vi "Is Name Multiplatform_Allow Multibyte.vi"(8 "error in (no error)":errorcluster, 9 "Replacement":string="-", 10 "name must work for all platforms (F)":bool, 11 "filename":string) -> (0 "error out":errorcluster, 1 "name had problem":bool, 3 "suggested filename":string, 4 "problem description":string)   [LabVIEW 2020, in "NI_Multibyte Utilities.lvlib"]
uses:
  <vilib>/Utility/Multibyte/NI_Multibyte Utilities.lvlib
panel:
  in  "Last Character Windows Warning":string="Windows filenames cannot terminate with the . character."
  in  "Platform Warnings":string[](array[string])=["Windows filenames cannot contain any of these characters: \\ : / * ? \" < > |.", "Macintosh filenames cannot contain the : character.", "Linux filenames cannot contain the / character."]
  in  "Empty filename":string="An empty string is not a valid filename."
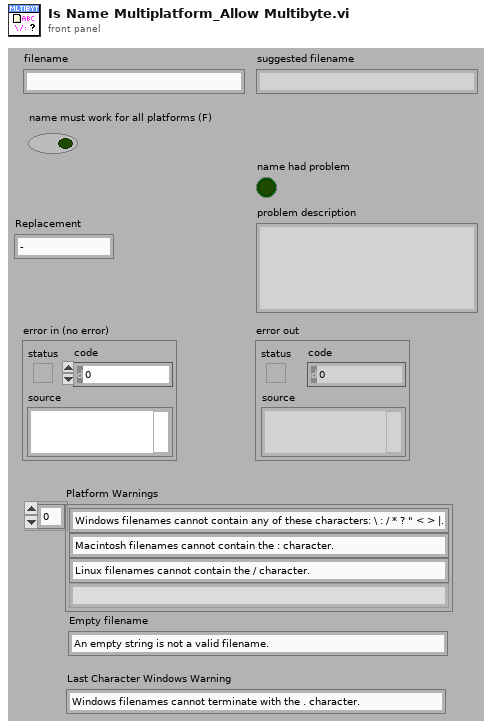
[diagram p1: front panel]
types:
  T1 = cluster{enum32{"invalid OS target", "Mac OS", "Windows 3.1", "Windows 95/NT", "Solaris 1", "Solaris 2", "HP-UX", "PowerMAX", "Linux", "Irix", "Rhapsody", "BeOS", "AIX", "OSF1", "VxWorks", "PharLap", "Carbon", "RTX", "Windows x64", "Linux x64"}[]}[]
  T2 = enum32{"invalid OS target", "Mac OS", "Windows 3.1", "Windows 95/NT", "Solaris 1", "Solaris 2", "HP-UX", "PowerMAX", "Linux", "Irix", "Rhapsody", "BeOS", "AIX", "OSF1", "VxWorks", "PharLap", "Carbon", "RTX", "Windows x64", "Linux x64", "Mac OS X x64"}
  T3 = enum32{"invalid OS target", "Mac OS", "Windows 3.1", "Windows 95/NT", "Solaris 1", "Solaris 2", "HP-UX", "PowerMAX", "Linux", "Irix", "Rhapsody", "BeOS", "AIX", "OSF1", "VxWorks", "PharLap", "Carbon", "RTX", "Windows x64", "Linux x64"}[]
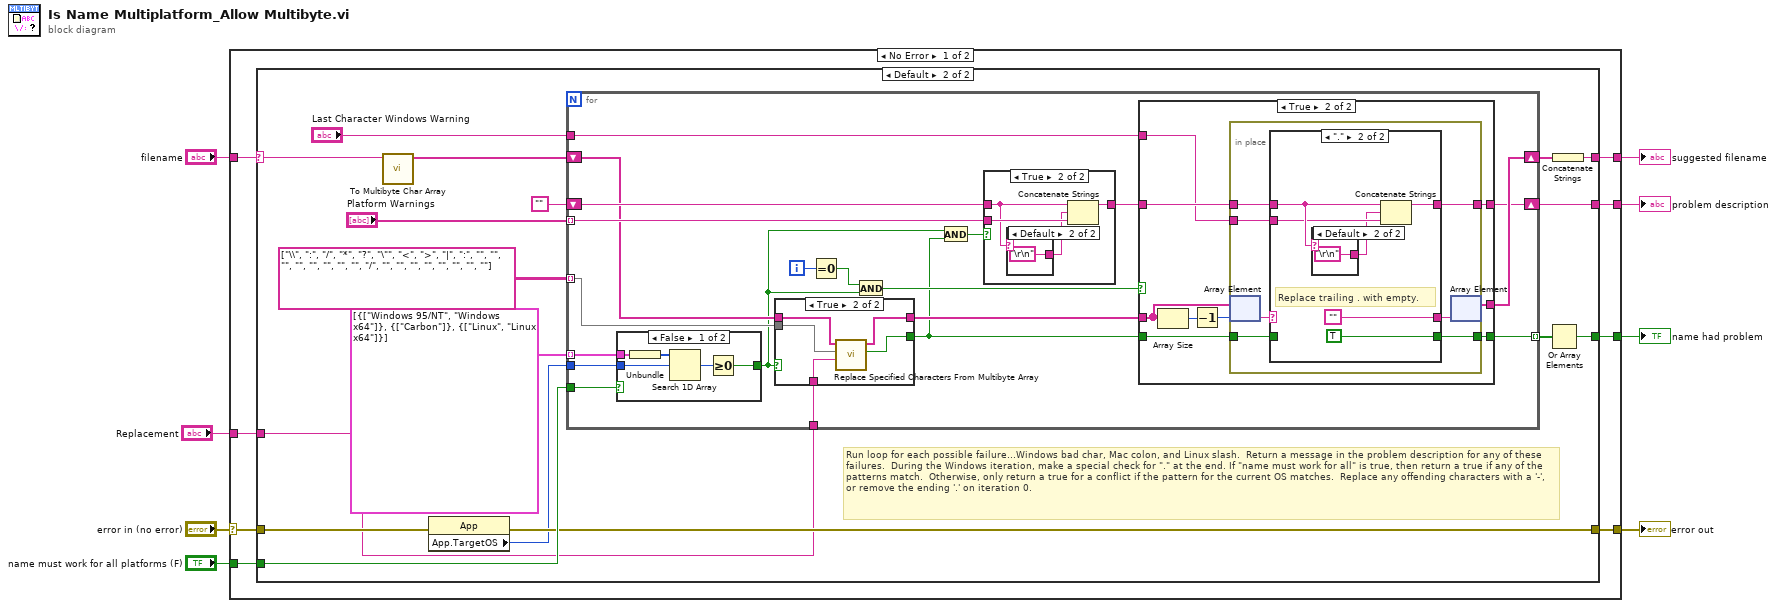
[diagram p0: block diagram]
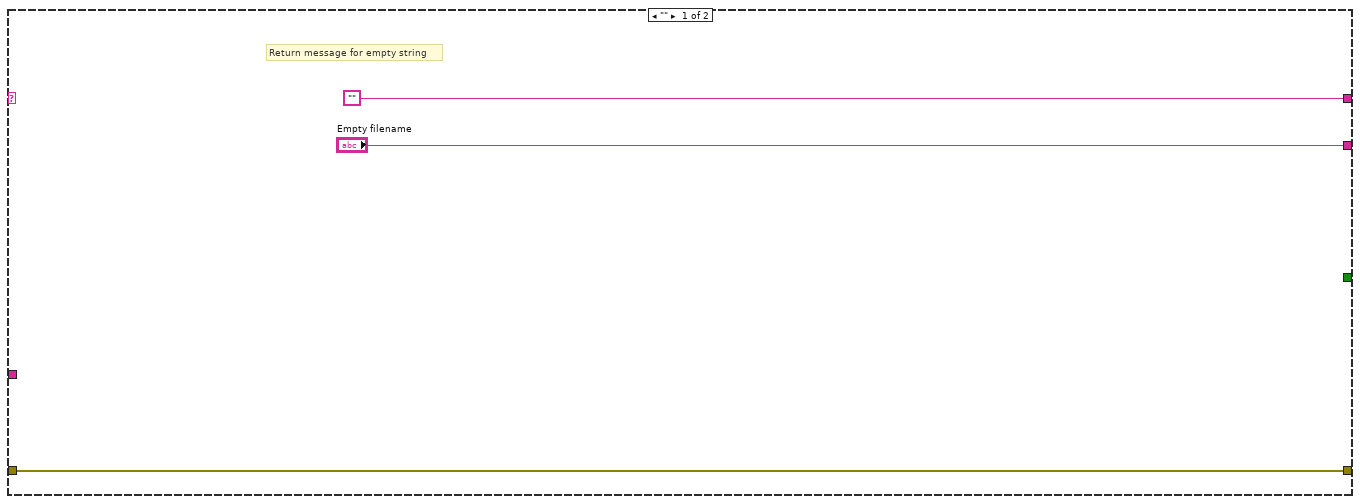
[diagram p2: hidden frame]
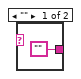
[diagram p5: hidden frame]
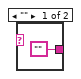
[diagram p9: hidden frame]
diagram:
  n1 = case shown="No Error" "error in (no error)" {
    selector: "error in (no error)" -> [w10 w106]
    tunnel: [w16 _] -> w8
    tunnel: [w15 _] -> w7
    tunnel: [w14 _] -> w6
    tunnel: "filename" -> [w13 _]
    tunnel: "name must work for all platforms (F)" -> [w12 _]
    tunnel: [w11 w106] -> w2
    tunnel: "Replacement" -> [w9 _]
    frame No Error {
      n2 = case shown="Default" w13 {
        selector: w13 -> [_ w25]
        tunnel: [_ w36] -> w16
        tunnel: ["Empty filename" w35] -> w15
        tunnel: ["" w22] -> w14
        tunnel: w12 -> [_ w33]
        tunnel: [w18 w32] -> w11
        tunnel: w10 -> [w18 w31]
        tunnel: w9 -> [_ w20]
        frame "" {
          # "Return message for empty string"
        }
        frame Default {
          # "Run loop for each possible failure...Windows bad char, Mac colon, and Linux slash.  Return a message in the problem description for any of these failures.  During the Windows iteration, make a special check for \".\" at the end. If \"name must work for all\" is true, then return a true if any of the patterns match.  Otherwise, only return a true for a conflict if the pattern for the current OS matches.  Replace any offending characters with a '-', or remove the ending '.' on iteration 0."
          n3 = call <vilib>:"To Multibyte Char Array.vi"("String"=w25) -> ("Array of Multibyte Chars"=w24:string[])  [unwired: 10 in]
          n4 = property class="App"(error in=w31) -> (error out=w32:errorcluster, "App.TargetOS"=w27:T2)  [unwired: 1 in, 1 out]
          n5 = for {
            tunnel: string[][] [["\\", ":", "/", "*", "?", "\"", "<", ">", "|"], [":", "", "", "", "", "", "", "", ""], ["/", "", "", "", "", "", "", "", ""]] -> [w50] mode=indexing
            shift-right: [w42] -> w35
            shift-left: "" -> [w56]
            tunnel: "Platform Warnings" -> [w55] mode=indexing
            tunnel: T1 [{[enum."Windows 95/NT", enum."Windows x64"]}, {[enum."Carbon"]}, {[enum."Linux", enum."Linux x64"]}] -> [w54] mode=indexing
            tunnel: w27 -> [w53]
            tunnel: w33 -> [w52]
            shift-right: [w45] -> w34
            shift-left: w24 -> [w51]
            tunnel: [w44] -> w26 mode=indexing
            tunnel: "Last Character Windows Warning" -> [w41]
            tunnel: w20 -> [w37]
            i -> [w49]
            n6 = case shown="False" w52 {
              selector: w52 -> [_ w98]
              tunnel: w54 -> [w97 _]
              tunnel: w53 -> [w95 _]
              tunnel: [w93 w98] -> w39
              frame False {
                n7 = Unbundle(w97) -> (w96:T3)
                n8 = Search 1D Array(1D array=w96, element=w95) -> (index of element=w94:i32)  [unwired: 1 out]
                n9 = Greater Or Equal To 0?(x=w94) -> (x >= 0?=w93:bool)
              }
              frame True {
              }
            }
            n10 = case shown="True" w39 {
              tunnel: w51 -> [w87 w92]
              tunnel: [w87 w91] -> w46
              tunnel: [_ w90] -> w38
              tunnel: w50 -> [_ w89]
              tunnel: w37 -> [_ w88]
              frame False {
              }
              frame True {
                n11 = call <vilib>:"Replace Specified Characters From Multibyte Array.vi"("Replacement"=w88, "Problem Characters"=w89, "Array of Multibyte Characters"=w92) -> ("Any Characters Removed?"=w90:bool, "Modified Array"=w91:string[])  [unwired: 6 in, 1 out]
              }
            }
            n12 = Equal To 0?(x=w49) -> (x = 0?=w48:bool)
            n13 = And(x=w48, y=w39) -> (x .and. y?=w47:bool)
            n14 = And(x=w39, y=w38) -> (x .and. y?=w40:bool)
            n15 = case shown="True" w40 {
              tunnel: w56 -> [w99 w101]
              tunnel: w55 -> [_ w102]
              tunnel: [w99 w103] -> w43
              frame False {
              }
              frame True {
                n16 = case shown="Default" w101 {
                  tunnel: ["" "\r\n"] -> w100
                  frame "" {
                  }
                  frame Default {
                  }
                }
                n17 = Concatenate Strings(w101, w100, w102) -> (w103:string)
              }
            }
            n18 = case shown="True" w47 {
              tunnel: w38 -> [w58 w63]
              tunnel: w46 -> [w59 w66]
              tunnel: [w59 w65] -> w45
              tunnel: [w58 w64] -> w44
              tunnel: w43 -> [w57 w62]
              tunnel: [w57 w61] -> w42
              tunnel: w41 -> [_ w60]
              frame False {
              }
              frame True {
                n19 = Array Size(array=w66) -> (size(s)=w68:i32)
                n20 = Decrement(x=w68) -> (x-1=w67:i32)
                n21 = in-place {
                  in-place-border: [w73] -> w64
                  in-place-border: w63 -> [w72]
                  in-place-border: w62 -> [w71]
                  in-place-border: [w70] -> w61
                  in-place-border: w60 -> [w69]
                  n22 = in-place-array #1(w66, w67) -> (w75:string)
                  n23 = case shown="\".\"" w75 {
                    selector: w75 -> [w78 _]
                    tunnel: [w78 ""] -> w74
                    tunnel: [w77 TRUE] -> w73
                    tunnel: w72 -> [w77 _]
                    tunnel: w71 -> [w76 w83]
                    tunnel: [w76 w82] -> w70
                    tunnel: w69 -> [_ w81]
                    frame Default {
                    }
                    frame "." {
                      # "Replace trailing . with empty."
                      n24 = case shown="Default" w83 {
                        tunnel: ["" "\r\n"] -> w80
                        frame "" {
                        }
                        frame Default {
                        }
                      }
                      n25 = Concatenate Strings(w83, w80, w81) -> (w82:string)
                    }
                  }
                  n26 = in-place-array #1(w74) -> (w65:string[])  [unwired: 1 out]
                }
              }
            }
          }
          n27 = Or Array Elements(Boolean array=w26) -> (logical OR=w36:bool)
          n28 = Concatenate Strings(w34) -> (w22:string)
        }
      }
    }
    frame Error {
    }
  }
  "problem description" <- w7
  "name had problem" <- w8
  "suggested filename" <- w6
  "error out" <- w2
